vi "X_Y_movePID_map.vi"() -> ()   [LabVIEW 2021]
doc: "Shows how to move a motor to an absolute position."
panel:
  out "return value (INIT)":dbl[](array[numeric])
  in  "Init_stop":bool
  in  "Position X":dbl
  in  "Home 4":bool
  in  "Position Y":dbl
  in  "Home 3":bool
  out "element 2":dbl
  in  "Home 2":bool
  in  "Y_HWSerialNum":i32=83828425
  in  "MG17Motor 2":refnum<k7>(container)
  out "element":dbl
  out "return value (PID)":dbl[](array[numeric])
  in  "X_HWSerialNum":i32=83828425
  in  "MG17Motor":refnum<k7>(container)
  in  "PID_Stop":bool
  in  "Home":bool
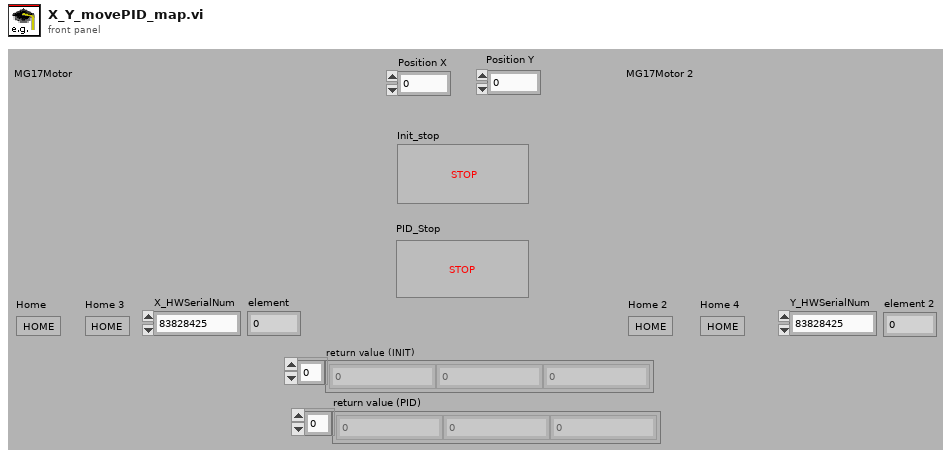
[diagram p1: front panel]
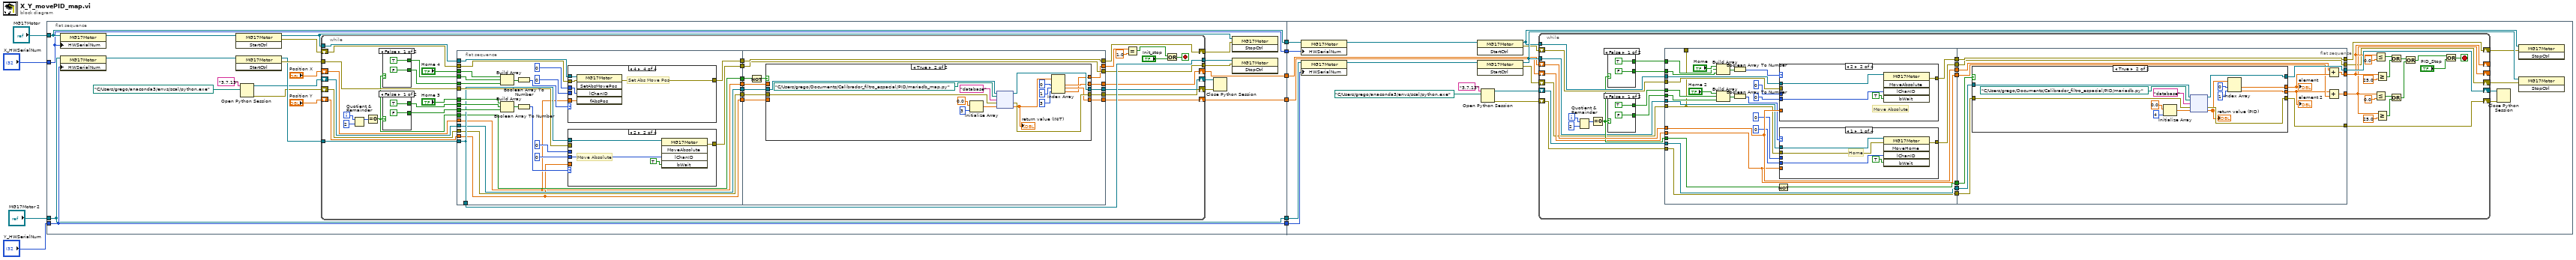
[diagram p0: block diagram]
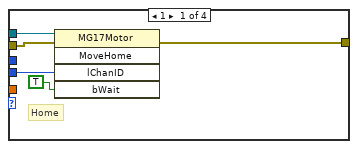
[diagram p2: hidden frame]
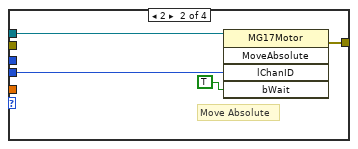
[diagram p3: hidden frame]
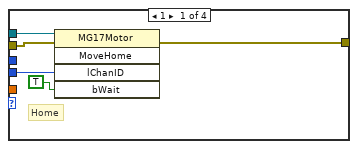
[diagram p5: hidden frame]
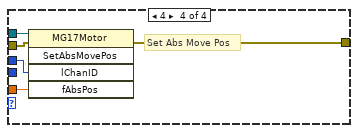
[diagram p7: hidden frame]
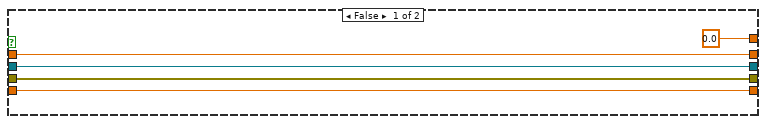
[diagram p8: hidden frame]
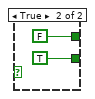
[diagram p9: hidden frame]
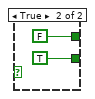
[diagram p10: hidden frame]
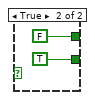
[diagram p11: hidden frame]
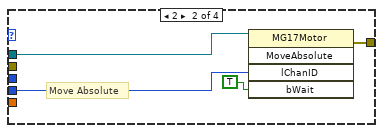
[diagram p12: hidden frame]
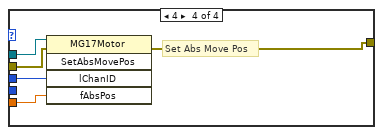
[diagram p14: hidden frame]
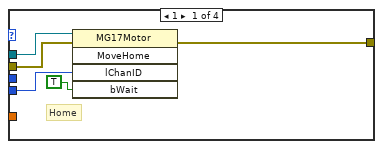
[diagram p15: hidden frame]
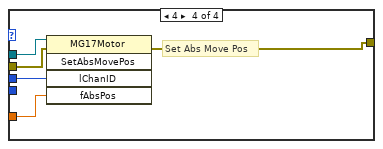
[diagram p17: hidden frame]
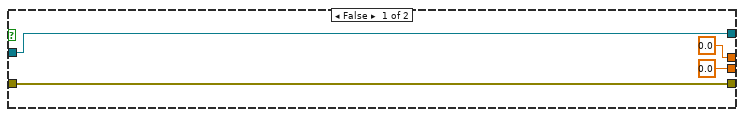
[diagram p18: hidden frame]
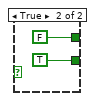
[diagram p19: hidden frame]
diagram:
  n1 = flat-sequence {
    tunnel: "MG17Motor 2" -> [w23]
    tunnel: "Y_HWSerialNum" -> [w24]
    tunnel: "MG17Motor" -> [w22]
    tunnel: "X_HWSerialNum" -> [w21]
    tunnel: [w24] -> w6
    tunnel: [w23] -> w5
    tunnel: [w22] -> w4
    tunnel: [w21] -> w3
    tunnel: [w16] -> w2
    tunnel: [w15] -> w1
    tunnel: w6 -> [w174]
    tunnel: w5 -> [w175]
    tunnel: w4 -> [w171]
    tunnel: w3 -> [w170]
    tunnel: w2 -> [w168]
    tunnel: w1 -> [w169]
    frame #0 {
      n2 = property class="MG17Motor"(reference=w22, "HWSerialNum"=w21) -> (reference out=w31:refnum<k7>)  [unwired: 1 in, 1 out]
      n3 = property class="MG17Motor"(reference=w23, "HWSerialNum"=w24) -> (reference out=w33:refnum<k7>)  [unwired: 1 in, 1 out]
      n4 = invoke class="MG17Motor" method="StartCtrl"(reference=w31) -> (reference out=w27:refnum<k7>, error out=w25:errorcluster)  [unwired: 2 in, 1 out]
      n5 = invoke class="MG17Motor" method="StartCtrl"(reference=w33) -> (reference out=w28:refnum<k7>, error out=w29:errorcluster)  [unwired: 2 in, 1 out]
      n6 = Open Python Session(python version="3.7.13" ("Python version"), python path=path "C:/Users/grego/anaconda3/envs/scal/python.exe" ("Python path")) -> (session out=w11:refnum<k35>, error out=w12:errorcluster)  [unwired: 1 in]
      n7 = while {
        tunnel: w29 -> [w66]
        tunnel: w28 -> [w65]
        tunnel: w27 -> [w64]
        shift-right: [w63] -> w26
        shift-left: w25 -> [w62]
        tunnel: [w53] -> w20
        tunnel: [w45] -> w19
        shift-right: [w50] -> w16
        shift-left: "Position Y" -> [w69]
        shift-right: [w49] -> w15
        shift-left: "Position X" -> [w67]
        shift-right: [w41] -> w14
        shift-left: w11 -> [w39]
        shift-right: [w42] -> w13
        shift-left: w12 -> [w40]
        i -> [w55]
        stop <- w34 stop-if-true
        n8 = Quotient & Remainder(x=w55, y=2) -> (x-y*floor(x/y)=w57:i32)  [unwired: 1 out]
        n9 = Equal To 0?(x=w57) -> (x = 0?=w48:bool)
        n10 = case shown="False" w48 {
          tunnel: [TRUE FALSE] -> w61
          tunnel: [FALSE TRUE] -> w60
          frame False {
          }
          frame True {
          }
        }
        n11 = case shown="False" w48 {
          tunnel: [TRUE FALSE] -> w59
          tunnel: [FALSE TRUE] -> w58
          frame False {
          }
          frame True {
          }
        }
        n12 = flat-sequence {
          tunnel: "Home 3" -> [w95]
          tunnel: w69 -> [w72]
          tunnel: "Home 4" -> [w90]
          tunnel: w67 -> [w71]
          tunnel: w66 -> [w85]
          tunnel: w65 -> [w77]
          tunnel: w64 -> [w84]
          tunnel: w62 -> [w82]
          tunnel: w61 -> [w81]
          tunnel: w60 -> [w80]
          tunnel: w59 -> [w79]
          tunnel: w58 -> [w78]
          tunnel: [w83] -> w54
          tunnel: [w77] -> w53
          tunnel: w39 -> [w76]
          tunnel: [w76] -> w52
          tunnel: w40 -> [w75]
          tunnel: [w75] -> w51
          tunnel: w48 -> [w74]
          tunnel: [w74] -> w47
          tunnel: [w73] -> w46
          tunnel: [w72] -> w44
          tunnel: [w71] -> w43
          tunnel: [w138] -> w63
          tunnel: w54 -> [w138]
          tunnel: w52 -> [w137]
          tunnel: w51 -> [w136]
          tunnel: [w135] -> w50
          tunnel: [w134] -> w49
          tunnel: w47 -> [w132]
          tunnel: [w131] -> w45
          tunnel: w46 -> [w131]
          tunnel: w44 -> [w130]
          tunnel: w43 -> [w129]
          tunnel: [w128] -> w42
          tunnel: [w127] -> w41
          tunnel: [w126] -> w38
          frame #0 {
            n13 = Build Array(w90, w81, w80) -> (w87:bool[])
            n14 = Build Array(w95, w79, w78) -> (w92:bool[])
            n15 = Boolean Array To Number(Boolean array=w87) -> (number=w88:u32)
            n16 = Boolean Array To Number(Boolean array=w92) -> (number=w93:u32)
            n17 = case shown="4" w88 {
              tunnel: w84 -> [w100 w104 _ w109]
              tunnel: 0 ("lChanID") -> [w99 w103 _ _]
              tunnel: w71 -> [_ _ _ w108]
              tunnel: [w98 w102 w105 w106] -> w83
              tunnel: w82 -> [w97 _ w105 w110]
              tunnel: 0 ("lChanID") -> [_ _ _ w107]
              frame 1 {
                # "Home"
                n18 = invoke class="MG17Motor" method="MoveHome"(reference=w100, error in=w97, "lChanID"=w99, "bWait"=TRUE) -> (error out=w98:errorcluster)  [unwired: 1 in, 4 out]
              }
              frame 2 {
                # "Move Absolute"
                n19 = invoke class="MG17Motor" method="MoveAbsolute"(reference=w104, "lChanID"=w103, "bWait"=TRUE) -> (error out=w102:errorcluster)  [unwired: 2 in, 4 out]
              }
              frame Default {
              }
              frame 4 {
                # "Set Abs Move Pos"
                n20 = invoke class="MG17Motor" method="SetAbsMovePos"(reference=w109, error in=w110, "lChanID"=w107, "fAbsPos"=w108) -> (error out=w106:errorcluster)  [unwired: 1 in, 4 out]
              }
            }
            n21 = case shown="2" w93 {
              tunnel: w77 -> [w115 w119 _ w124]
              tunnel: 0 ("lChanID") -> [w114 w118 _ _]
              tunnel: w72 -> [_ _ _ w123]
              tunnel: [w113 w117 w120 w121] -> w73
              tunnel: w85 -> [w112 _ w120 w125]
              tunnel: 0 ("lChanID") -> [_ _ _ w122]
              frame 1 {
                # "Home"
                n22 = invoke class="MG17Motor" method="MoveHome"(reference=w115, error in=w112, "lChanID"=w114, "bWait"=TRUE) -> (error out=w113:errorcluster)  [unwired: 1 in, 4 out]
              }
              frame 2 {
                # "Move Absolute"
                n23 = invoke class="MG17Motor" method="MoveAbsolute"(reference=w119, "lChanID"=w118, "bWait"=TRUE) -> (error out=w117:errorcluster)  [unwired: 2 in, 4 out]
              }
              frame Default {
              }
              frame 4 {
                # "Set Abs Move Pos"
                n24 = invoke class="MG17Motor" method="SetAbsMovePos"(reference=w124, error in=w125, "lChanID"=w122, "fAbsPos"=w123) -> (error out=w121:errorcluster)  [unwired: 1 in, 4 out]
              }
            }
          }
          frame #1 {
            n25 = Not(x=w132) -> (.not. x?=w133:bool)
            n26 = case shown="True" w133 {
              tunnel: w137 -> [w143 w149]
              tunnel: w136 -> [w142 w148]
              tunnel: [w143 w154] -> w127
              tunnel: [w142 w153] -> w128
              tunnel: [w140 w150] -> w134
              tunnel: [w141 w146] -> w135
              tunnel: w130 -> [w141 _]
              tunnel: w129 -> [w140 _]
              tunnel: [0.0 ("element") w144] -> w126
              frame False {
              }
              frame True {
                n27 = Initialize Array(0.0 ("element"), 3 ("dimension size")) -> (w158:dbl[])
                n28 = node(w149, path "C:/Users/grego/Documents/Calibrador_filtro_espacial/PID/mariadb_map.py" ("module path"), "database" ("function name"), w148, w158) -> (w154:refnum<k35>, w153:errorcluster, w152:dbl[])  [unwired: 2 out]
                "return value (INIT)" <- w152
                n29 = Index Array(array=w152, index #1=0 ("index"), index #2=1 ("index"), index #3=3 ("index")) -> (element #1=w150:dbl, element #2=w146:dbl, element #3=w144:dbl)
              }
            }
          }
        }
        n30 = Equal?(x=w38, y=1.0) -> (x = y?=w36:bool)
        n31 = Or(x=w36, y="Init_stop") -> (x .or. y?=w34:bool)
      }
      n32 = Close Python Session(session in=w14, error in=w13) -> ()  [unwired: 1 out]
      n33 = invoke class="MG17Motor" method="StopCtrl"(reference=w27, error in=w26) -> ()  [unwired: 1 in, 3 out]
      n34 = invoke class="MG17Motor" method="StopCtrl"(reference=w20, error in=w19) -> ()  [unwired: 1 in, 3 out]
    }
    frame #1 {
      n35 = property class="MG17Motor"(reference=w171, "HWSerialNum"=w170) -> (reference out=w179:refnum<k7>)  [unwired: 1 in, 1 out]
      n36 = property class="MG17Motor"(reference=w175, "HWSerialNum"=w174) -> (reference out=w184:refnum<k7>)  [unwired: 1 in, 1 out]
      n37 = invoke class="MG17Motor" method="StartCtrl"(reference=w179) -> (reference out=w176:refnum<k7>, error out=w177:errorcluster)  [unwired: 2 in, 1 out]
      n38 = invoke class="MG17Motor" method="StartCtrl"(reference=w184) -> (reference out=w186:refnum<k7>, error out=w187:errorcluster)  [unwired: 2 in, 1 out]
      n39 = Open Python Session(python version="3.7.13" ("Python version"), python path=path "C:/Users/grego/anaconda3/envs/scal/python.exe" ("Python path")) -> (session out=w180:refnum<k35>, error out=w181:errorcluster)  [unwired: 1 in]
      n40 = while {
        shift-left: w177 -> [w227]
        shift-right: [w228] -> w178
        tunnel: w176 -> [w229]
        shift-right: [w210] -> _
        shift-left: w169 -> [w221]
        shift-right: [w218] -> w182
        shift-left: w180 -> [w215]
        shift-right: [w217] -> w183
        shift-left: w181 -> [w213]
        tunnel: w186 -> [w203]
        shift-right: [w193] -> _
        shift-left: w168 -> [w200]
        shift-right: [w192] -> w185
        shift-left: w187 -> [w190]
        i -> [w225]
        stop <- w191 stop-if-true
        n41 = Quotient & Remainder(x=w225, y=2) -> (x-y*floor(x/y)=w226:i32)  [unwired: 1 out]
        n42 = Equal To 0?(x=w226) -> (x = 0?=w204:bool)
        n43 = case shown="False" w204 {
          tunnel: [TRUE FALSE] -> w223
          tunnel: [FALSE TRUE] -> w222
          frame False {
          }
          frame True {
          }
        }
        n44 = case shown="False" w204 {
          tunnel: [TRUE FALSE] -> w202
          tunnel: [FALSE TRUE] -> w201
          frame False {
          }
          frame True {
          }
        }
        n45 = flat-sequence {
          tunnel: w229 -> [w258]
          tunnel: w227 -> [w255]
          tunnel: w223 -> [w238]
          tunnel: w222 -> [w237]
          tunnel: w221 -> [w247]
          tunnel: w204 -> [w251]
          tunnel: [w256] -> w220
          tunnel: [w250] -> w219
          tunnel: [w249] -> w216
          tunnel: w215 -> [w249]
          tunnel: [w248] -> w214
          tunnel: w213 -> [w248]
          tunnel: [w247] -> w212
          tunnel: w203 -> [w246]
          tunnel: [w234] -> _
          tunnel: w202 -> [w244]
          tunnel: w201 -> [w243]
          tunnel: w200 -> [w235]
          tunnel: [w236] -> w199
          tunnel: [w235] -> w198
          tunnel: w190 -> [w234]
          tunnel: [w302] -> w228
          tunnel: w220 -> [w302]
          tunnel: w219 -> [w299]
          tunnel: [w301] -> w218
          tunnel: [w300] -> w217
          tunnel: [w296] -> w210
          tunnel: w216 -> [w297]
          tunnel: w214 -> [w298]
          tunnel: w212 -> [w295]
          tunnel: w199 -> [w290]
          tunnel: w198 -> [w293]
          tunnel: [w292] -> w193
          tunnel: [w290] -> w192
          frame #0 {
            n46 = Build Array("Home", w238, w237) -> (w253:bool[])
            n47 = Build Array("Home 2", w244, w243) -> (w242:bool[])
            n48 = Boolean Array To Number(Boolean array=w253) -> (number=w254:u32)
            n49 = Boolean Array To Number(Boolean array=w242) -> (number=w241:u32)
            n50 = Not(x=w251) -> (.not. x?=w250:bool)
            n51 = case shown="2" w254 {
              tunnel: w258 -> [w279 w283 _ w288]
              tunnel: 0 ("lChanID") -> [w278 w282 _ _]
              tunnel: w247 -> [_ _ _ w287]
              tunnel: [w277 w281 w284 w285] -> w256
              tunnel: w255 -> [w276 _ w284 w289]
              tunnel: 0 ("lChanID") -> [_ _ _ w286]
              frame 1 {
                # "Home"
                n52 = invoke class="MG17Motor" method="MoveHome"(reference=w279, error in=w276, "lChanID"=w278, "bWait"=TRUE) -> (error out=w277:errorcluster)  [unwired: 1 in, 4 out]
              }
              frame 2 {
                # "Move Absolute"
                n53 = invoke class="MG17Motor" method="MoveAbsolute"(reference=w283, "lChanID"=w282, "bWait"=TRUE) -> (error out=w281:errorcluster)  [unwired: 2 in, 4 out]
              }
              frame Default {
              }
              frame 4 {
                # "Set Abs Move Pos"
                n54 = invoke class="MG17Motor" method="SetAbsMovePos"(reference=w288, error in=w289, "lChanID"=w286, "fAbsPos"=w287) -> (error out=w285:errorcluster)  [unwired: 1 in, 4 out]
              }
            }
            n55 = case shown="1" w241 {
              tunnel: w246 -> [w264 w268 _ w273]
              tunnel: 0 ("lChanID") -> [w263 w267 _ _]
              tunnel: w235 -> [_ _ _ w272]
              tunnel: [w262 w266 w269 w270] -> w236
              tunnel: w234 -> [w261 _ w269 w274]
              tunnel: 0 ("lChanID") -> [_ _ _ w271]
              frame 1 {
                # "Home"
                n56 = invoke class="MG17Motor" method="MoveHome"(reference=w264, error in=w261, "lChanID"=w263, "bWait"=TRUE) -> (error out=w262:errorcluster)  [unwired: 1 in, 4 out]
              }
              frame 2 {
                # "Move Absolute"
                n57 = invoke class="MG17Motor" method="MoveAbsolute"(reference=w268, "lChanID"=w267, "bWait"=TRUE) -> (error out=w266:errorcluster)  [unwired: 2 in, 4 out]
              }
              frame Default {
              }
              frame 4 {
                # "Set Abs Move Pos"
                n58 = invoke class="MG17Motor" method="SetAbsMovePos"(reference=w273, error in=w274, "lChanID"=w271, "fAbsPos"=w272) -> (error out=w270:errorcluster)  [unwired: 1 in, 4 out]
              }
            }
          }
          frame #1 {
            n59 = case shown="True" w299 {
              tunnel: w297 -> [w306 w310]
              tunnel: w298 -> [w305 w309]
              tunnel: [w306 w315] -> w301
              tunnel: [w305 w314] -> w300
              tunnel: [0.0 w311] -> w294
              tunnel: [0.0 ("element") w307] -> w291
              frame False {
              }
              frame True {
                n60 = Initialize Array(0.0 ("element"), 4 ("dimension size")) -> (w319:dbl[])
                n61 = node(w310, path "C:/Users/grego/Documents/Calibrador_filtro_espacial/PID/mariadb.py" ("module path"), "database" ("function name"), w309, w319) -> (w315:refnum<k35>, w314:errorcluster, w313:dbl[])  [unwired: 2 out]
                "return value (PID)" <- w313
                n62 = Index Array(array=w313, index #1=0 ("index"), index #2=1 ("index")) -> (element #1=w311:dbl, element #2=w307:dbl)
              }
            }
            "element" <- w294
            "element 2" <- w291
            n63 = Add(x=w295, y=w294) -> (x+y=w296:dbl)
            n64 = Add(x=w291, y=w293) -> (x+y=w292:dbl)
          }
        }
        n65 = Less Or Equal?(x=w210, y=0.0) -> (x <= y?=w208:bool)
        n66 = Less Or Equal?(x=w193, y=0.0) -> (x <= y?=w195:bool)
        n67 = Greater Or Equal?(x=w210, y=25.0) -> (x >= y?=w207:bool)
        n68 = Greater Or Equal?(x=w193, y=25.0) -> (x >= y?=w194:bool)
        n69 = Or(x=w208, y=w207) -> (x .or. y?=w205:bool)
        n70 = Or(x=w195, y=w194) -> (x .or. y?=w188:bool)
        n71 = Or(x=w205, y=w188) -> (x .or. y?=w206:bool)
        n72 = Or(x=w206, y="PID_Stop") -> (x .or. y?=w191:bool)
      }
      n73 = Close Python Session(session in=w182, error in=w183) -> ()  [unwired: 1 out]
      n74 = invoke class="MG17Motor" method="StopCtrl"(reference=w176, error in=w178) -> ()  [unwired: 1 in, 3 out]
      n75 = invoke class="MG17Motor" method="StopCtrl"(reference=w186, error in=w185) -> ()  [unwired: 1 in, 3 out]
    }
  }
